vi "E517_Sample_Application_1.vi"() -> ()   [LabVIEW 2011]
doc: "This VI demonstrates how to initialize an E-517 system, how to move one connected axis and how to query for the position value of this axis. \n\nIn this example the E-517 is connected through COM port 1 with baudrate 57600. The VI runs E517_Configuration_Setup.vi with these specified settings, moves the first connected axis relative to its current position and reads the position of this axis. The diagram shows how to combine the driver VIs for these tasks. \n\nWarning: Before running this VI, modify the \"Interface\" and \"RS232 settings\" (or \"TCP/IP settings\" or \"GPIB settings\" or \"USB settings\") to reflect your configuration. The predefined settings provided with the VI probably do not match your system."
panel:
  in  "stop":bool
  in  "error in":errorcluster
  out "Running":bool caption="E517_Configuration_Setup is running"
  out "error out":errorcluster
  out "Position Axis":dbl[](array[numeric]) format="%.6f"
  out "Conn. Axes":string[](array[string])
  out "Identification":string
  # "Simple E-517 sample program"
  # "This VI demonstrates how to statically define an E-517 configuration with one connected axis. In this example the E-517 is connected\nthrough COM port 1 with baudrate 57600. The VI runs E517_Configuration_Setup.vi with these specified settings, moves the axis to the\nmiddle position of its range and reads the position of the axis. The diagram shows how to combine the driver VIs for these tasks. \n\nWarning: Before running this VI, modify the \"Interface\" and \"RS232 settings\" to reflect your configuration. The predefined \n                 settings provided with the VI probably do not match your system."
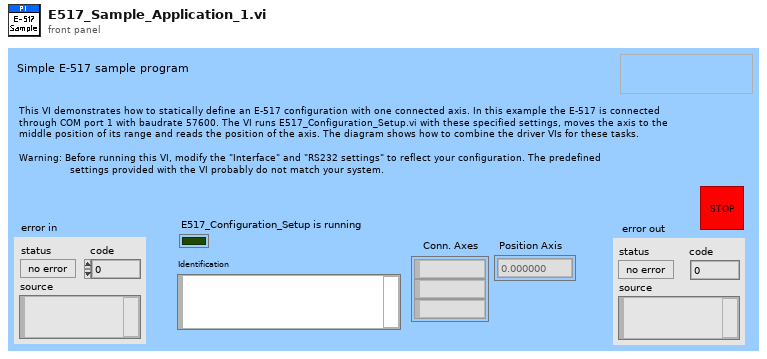
[diagram p1: front panel]
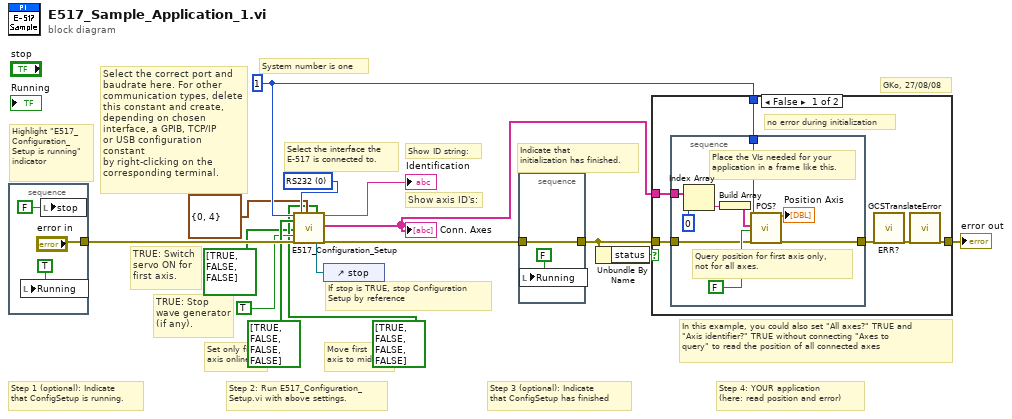
[diagram p0: block diagram]
diagram:
  w6 = u16 0 items=["RS232", "GPIB", "TCP/IP", "USB"] ("Interface")
  w14 = 1 ("System no.")
  # "Move first\naxis to middle."
  # "TRUE: Stop\nwave generator\n(if any)."
  # "In this example, you could also set \"All axes?\" TRUE and\n\"Axis identifier?\" TRUE without connecting \"Axes to \nquery\" to read the position of all connected axes"
  # "If stop is TRUE, stop Configuration\nSetup by reference"
  # "Set only first\naxis online."
  # "Select the interface the\nE-517 is connected to."
  # "Select the correct port and \nbaudrate here. For other \ncommunication types, delete\nthis constant and create, \ndepending on chosen \ninterface, a GPIB, TCP/IP \nor USB configuration constant\nby right-clicking on the \ncorresponding terminal."
  # "GKo, 27/08/08"
  # "Step 4: YOUR application\n(here: read position and error)"
  # "Step 3 (optional): Indicate\nthat ConfigSetup has finished"
  # "Step 2: Run E517_Configuration_\nSetup.vi with above settings."
  # "Step 1 (optional): Indicate\nthat ConfigSetup is running."
  # "Indicate that\ninitialization has finished."
  # "Highlight \"E517_\nConfiguration_\nSetup is running\"\nindicator"
  # "Show axis ID's:"
  # "Show ID string:"
  # "TRUE: Switch \nservo ON for\nfirst axis."
  # "System number is one"
  n1 = stacked-sequence {
    tunnel: ["error in"] -> w11
    frame #0 {
      n2 = local write "Running"(TRUE ("Running")) -> ()
      n3 = local write "stop"(FALSE ("stop")) -> ()
    }
  }
  n4 = control-ref of="stop"() -> (w7:refnum<vi>)
  n5 = call "E517_Configuration_Setup.vi"("System no."=w14, "Set channel online?"=bool[] [TRUE, FALSE, FALSE, FALSE] ("Are stages connected?"), "Switch servo on?"=bool[] [TRUE, FALSE, FALSE], "Stop wave generator\noutput (if any)"=TRUE ("All axes?"), "error in"=w11, "Interface"=w6, "RS232 settings"=cluster{"Portnumber":i32, "Baudrate":u16} {"Portnumber"=0, "Baudrate"=4}, "Axes to move to middle"=bool[] [TRUE, FALSE, FALSE, FALSE] ("Are stages connected?"), "Stop refnum"=w7) -> ("Identification"=→"Identification":string, "Conn. Axes"=w2:string[], "error out"=w12:errorcluster)  [unwired: 4 in, 4 out]
  "Conn. Axes" <- w2
  n6 = stacked-sequence {
    tunnel: w12 -> [w20]
    tunnel: [w20] -> w9
    frame #0 {
      n7 = local write "Running"(FALSE ("Running")) -> ()
    }
  }
  n8 = Unbundle By Name(w9) -> ("status"=w8:bool)
  n9 = case shown="False" w8 {
    tunnel: w14 -> [w26 _]
    tunnel: [w22 w36] -> w13
    tunnel: w9 -> [w25 w36]
    tunnel: w2 -> [w21 _]
    frame False {
      # "no error during initialization"
      n10 = stacked-sequence {
        tunnel: w26 -> [w35]
        tunnel: w25 -> [w32]
        tunnel: [w31] -> w24
        tunnel: w21 -> [w28]
        frame #0 {
          # "Place the VIs needed for your\napplication in a frame like this."
          # "Query position for first axis only,\nnot for all axes."
          n11 = Index Array(array=w28, index=0) -> (element=w30:string)
          n12 = Build Array(w30) -> (w29:string[])
          n13 = call "POS?.vi"("System no."=w35, "Axes to query"=w29, "All axes?"=FALSE, "error in"=w32) -> ("Position"=→"Position Axis":dbl[], "error out"=w31:errorcluster)  [unwired: 1 in, 13 out]
        }
      }
      n14 = call "ERR?.vi"("error in"=w24) -> ("error out"=w23:errorcluster)  [unwired: 1 in, 17 out]
      n15 = call "GCSTranslateError.vi"("error in"=w23) -> ("error out"=w22:errorcluster)  [unwired: 18 out]
    }
    frame True {
      # "Error during initialization,\nstop execution here."
    }
  }
  "error out" <- w13
